vi "ReadTSV.vi"(11 "Path":path) -> (2 "Complex FRF":cluster{dbl, "df":dbl, cdb[]}, 3 "all rows":dbl[][](array[numeric]))   [LabVIEW 2022 SP3]
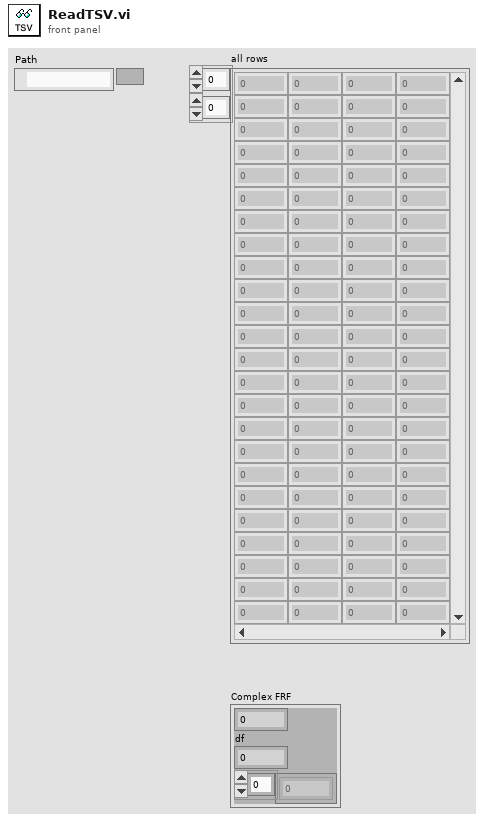
[diagram p1: front panel]
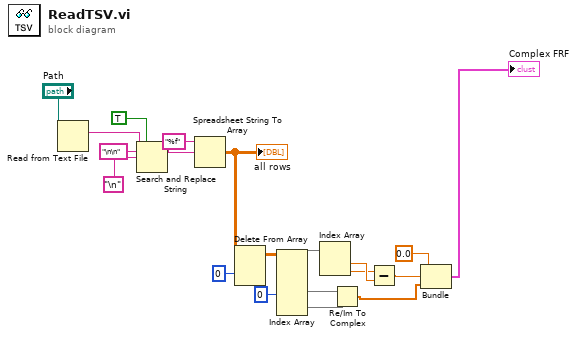
[diagram p0: block diagram]
diagram:
  n1 = Read from Text File(file (use dialog)="Path") -> (text=w2:string)  [unwired: 3 in, 3 out]
  n2 = Search and Replace String(replace all?=TRUE ("replace all? (F)"), input string=w2, search string="\n\n", replace string="\n" ("search string")) -> (result string=w6:string)  [unwired: 4 in, 3 out]
  n3 = Spreadsheet String To Array(format string="%f", spreadsheet string=w6) -> (array=w8:dbl[][])  [unwired: 2 in]
  "all rows" <- w8
  n4 = Delete From Array(array=w8, index (row)=0) -> (array with subset deleted=w10:dbl[][])  [unwired: 2 in, 1 out]
  n5 = Index Array(array=w10, index (col) #1=0 ("disabled index (col)")) -> (element #1=w11:dbl[], element #2=w19:dbl[], element #3=w20:dbl[])  [unwired: 5 in]
  n6 = Index Array(array=w11) -> (element #1=w13:dbl, element #2=w12:dbl)  [unwired: 2 in]
  n7 = Re/Im To Complex(1:w20, 2:w19) -> (0:w16:cdb[])
  n8 = Subtract(x=w12, y=w13) -> (x-y=w14:dbl)
  n9 = Bundle(0.0, w14, w16) -> (→"Complex FRF":cluster{dbl, dbl, cdb[]})  [unwired: 1 in]
